vi "zmq_libpath.vi"() -> (0 "path":path)   [LabVIEW 2020, in "zeromq.lvlib"]
doc: "Returns an absolute path to the LVZMQ shared library on the host system."
uses:
  zeromq.lvlib
panel:
  # "ØMQ"
  # "labview"
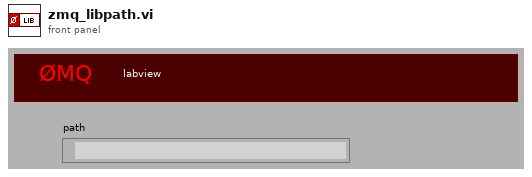
[diagram p1: front panel]
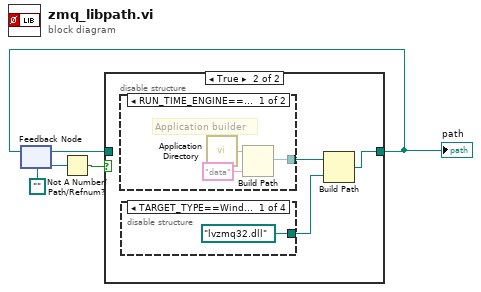
[diagram p0: block diagram]
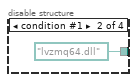
[diagram p3: hidden frame]
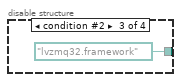
[diagram p4: hidden frame]
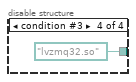
[diagram p5: hidden frame]
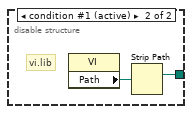
[diagram p6: hidden frame]
diagram:
  n1 = feedback #1(path "") -> (w2:path)
  n2 = Not A Number/Path/Refnum?(number/path/refnum=w2) -> (NaN/Path/Refnum?=w3:bool)
  n3 = case shown="True" w3 {
    tunnel: w2 -> [w5 _]
    tunnel: [w5 w6] -> w1
    frame False {
    }
    frame True {
      n4 = disable-structure shown="RUN_TIME_ENGINE==True" {
        disable-tunnel: [w15 w17] -> w8
        frame condition #0 {
          # "Application builder"
          n5 = call "Application Directory.vi"() -> ("Application Directory"=w13:path)
          n6 = Build Path(base path=w13, name or relative path="data") -> (appended path=w15:path)
        }
        frame condition #1 (active) {
          # "vi.lib"
          n7 = property class="VI"() -> ("Path"=w16:path)  [unwired: 2 in, 2 out]
          n8 = Strip Path(path=w16) -> (stripped path=w17:path)  [unwired: 1 out]
        }
      }
      n9 = disable-structure shown="TARGET_TYPE==Windows&&TARGET_BITNESS==32" {
        disable-tunnel: [path "lvzmq32.dll" ("appended path") path "lvzmq64.dll" ("appended path") path "lvzmq32.framework" ("appended path") path "lvzmq32.so" ("appended path")] -> w7
        frame condition #0 (active) {
        }
        frame condition #1 {
        }
        frame condition #2 {
        }
        frame condition #3 {
        }
      }
      n10 = Build Path(base path=w8, name or relative path=w7) -> (appended path=w6:path)
    }
  }
  "path" <- w1
  n11 = feedback-in #1(w1) -> ()
